vi "Ramp Generation SB.vi"() -> ()   [LabVIEW 2019]
panel:
  out "Ramp Output":waveform(dbl)(graph)
  in  "Time Span":dbl
  in  "# Points":dbl
  in  "Min":dbl
  in  "Max":dbl
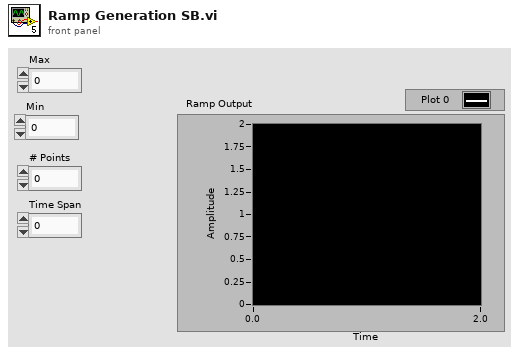
[diagram p1: front panel]
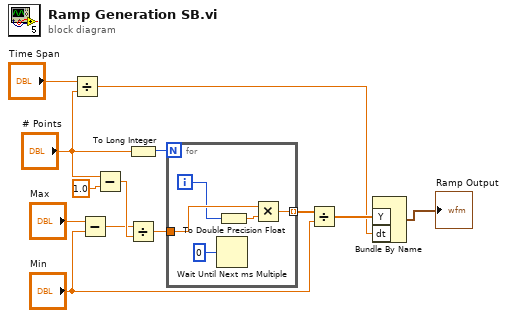
[diagram p0: block diagram]
diagram:
  n1 = Divide(x="Time Span", y="# Points") -> (x/y=w2:dbl)
  n2 = Subtract(x="Max", y="Min") -> (x-y=w10:dbl)
  n3 = Subtract(x="# Points", y=1.0) -> (x-y=w11:dbl)
  n4 = To Long Integer(number="# Points") -> (32bit integer=w8:i32)
  n5 = Divide(x=w10, y=w11) -> (x/y=w9:dbl)
  n6 = for {
    N: w8 -> [_]
    tunnel: w9 -> [w18]
    tunnel: [w14] -> w7 mode=indexing
    i -> [w17]
    n7 = Wait Until Next ms Multiple(millisecond multiple=u32 0) -> ()  [unwired: 1 out]
    n8 = To Double Precision Float(number=w17) -> (double precision float=w16:dbl)
    n9 = Multiply(x=w18, y=w16) -> (x*y=w14:dbl)
  }
  n10 = Divide(x=w7, y="Min") -> (x/y=w3:dbl[])
  n11 = Bundle By Name("Y"=w3, "dt"=w2) -> (→"Ramp Output":waveform(dbl))  [unwired: 1 in]
